vi "Write VISA Refnum.vi"(8 "error in":errorcluster, 10 "VISA Refnum in":refnum<visa-resource-name>, 11 "VISA Interface in":refnum<class "VISA Interface.lvclass">) -> (0 "error out":errorcluster, 3 "VISA Interface out":refnum<class "VISA Interface.lvclass">)   [LabVIEW 2020, in "Plugin Instrument Driver.lvlib" / "VISA Interface.lvclass"]
doc: "Write VISA Refnum"
uses:
  VISA Interface.lvclass
  VISA Interface.lvclass/VISA Interface.ctl
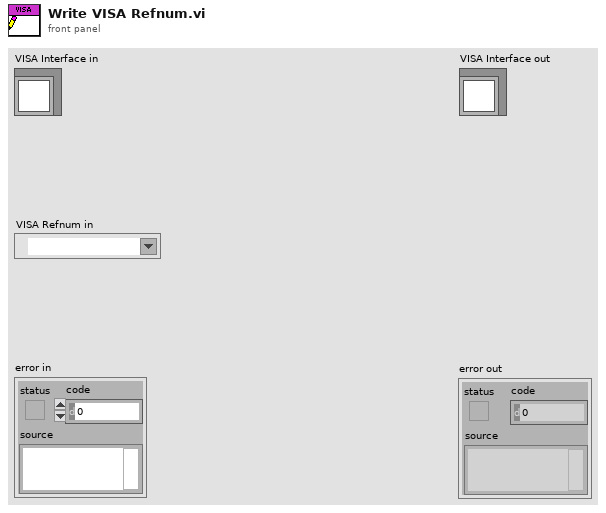
[diagram p1: front panel]
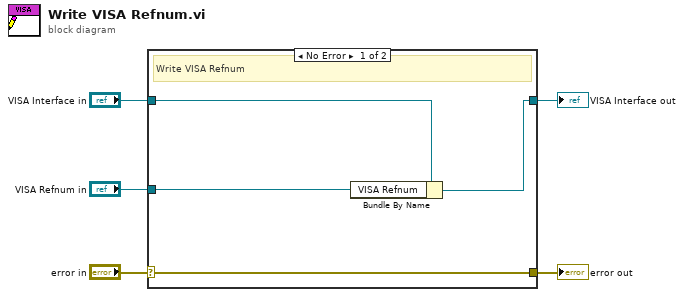
[diagram p0: block diagram]
diagram:
  n1 = case shown="No Error" "error in" {
    selector: "error in" -> [w9 w10]
    tunnel: [w9 w10] -> w4
    tunnel: [w7 w11] -> w2
    tunnel: "VISA Interface in" -> [w8 w11]
    tunnel: "VISA Refnum in" -> [w6 _]
    frame No Error {
      # "Write VISA Refnum"
      n2 = Bundle By Name(cluster=w8, "VISA Refnum"=w6) -> (w7:refnum<class "VISA Interface.lvclass">)
    }
    frame Error {
      # "Error Case"
    }
  }
  "error out" <- w4
  "VISA Interface out" <- w2
